vi "specify_roi.vi"(1 "input cluster":T3) -> (0 "output cluster":cluster{"Value":i32, dbl[], "Set":bool})   [LabVIEW 2015]
uses:
  <vilib>/vision/Avi1.llb/AviRefnum.ctl
  <vilib>/userdefined/High Color/IMAQdx.ctl
panel:
  in  "Store ROI from Coords":bool
  in  "Store ROI from image":bool
  in  "ROI Type":bool
  in  "ROI type flag":i32=-1
  in  "y2":i32
  in  "x2":i32
  in  "y1":i32
  in  "x1":i32
  out "initital frame number":i32
  in  "Reset":bool
  out "Image":T4(plugin-control)
  in  "Cancel":bool
  in  "Set":bool
  # "ROI Type"
  # "Rectangle"
  # "Ellipse"
  # "ROI Coordinates"
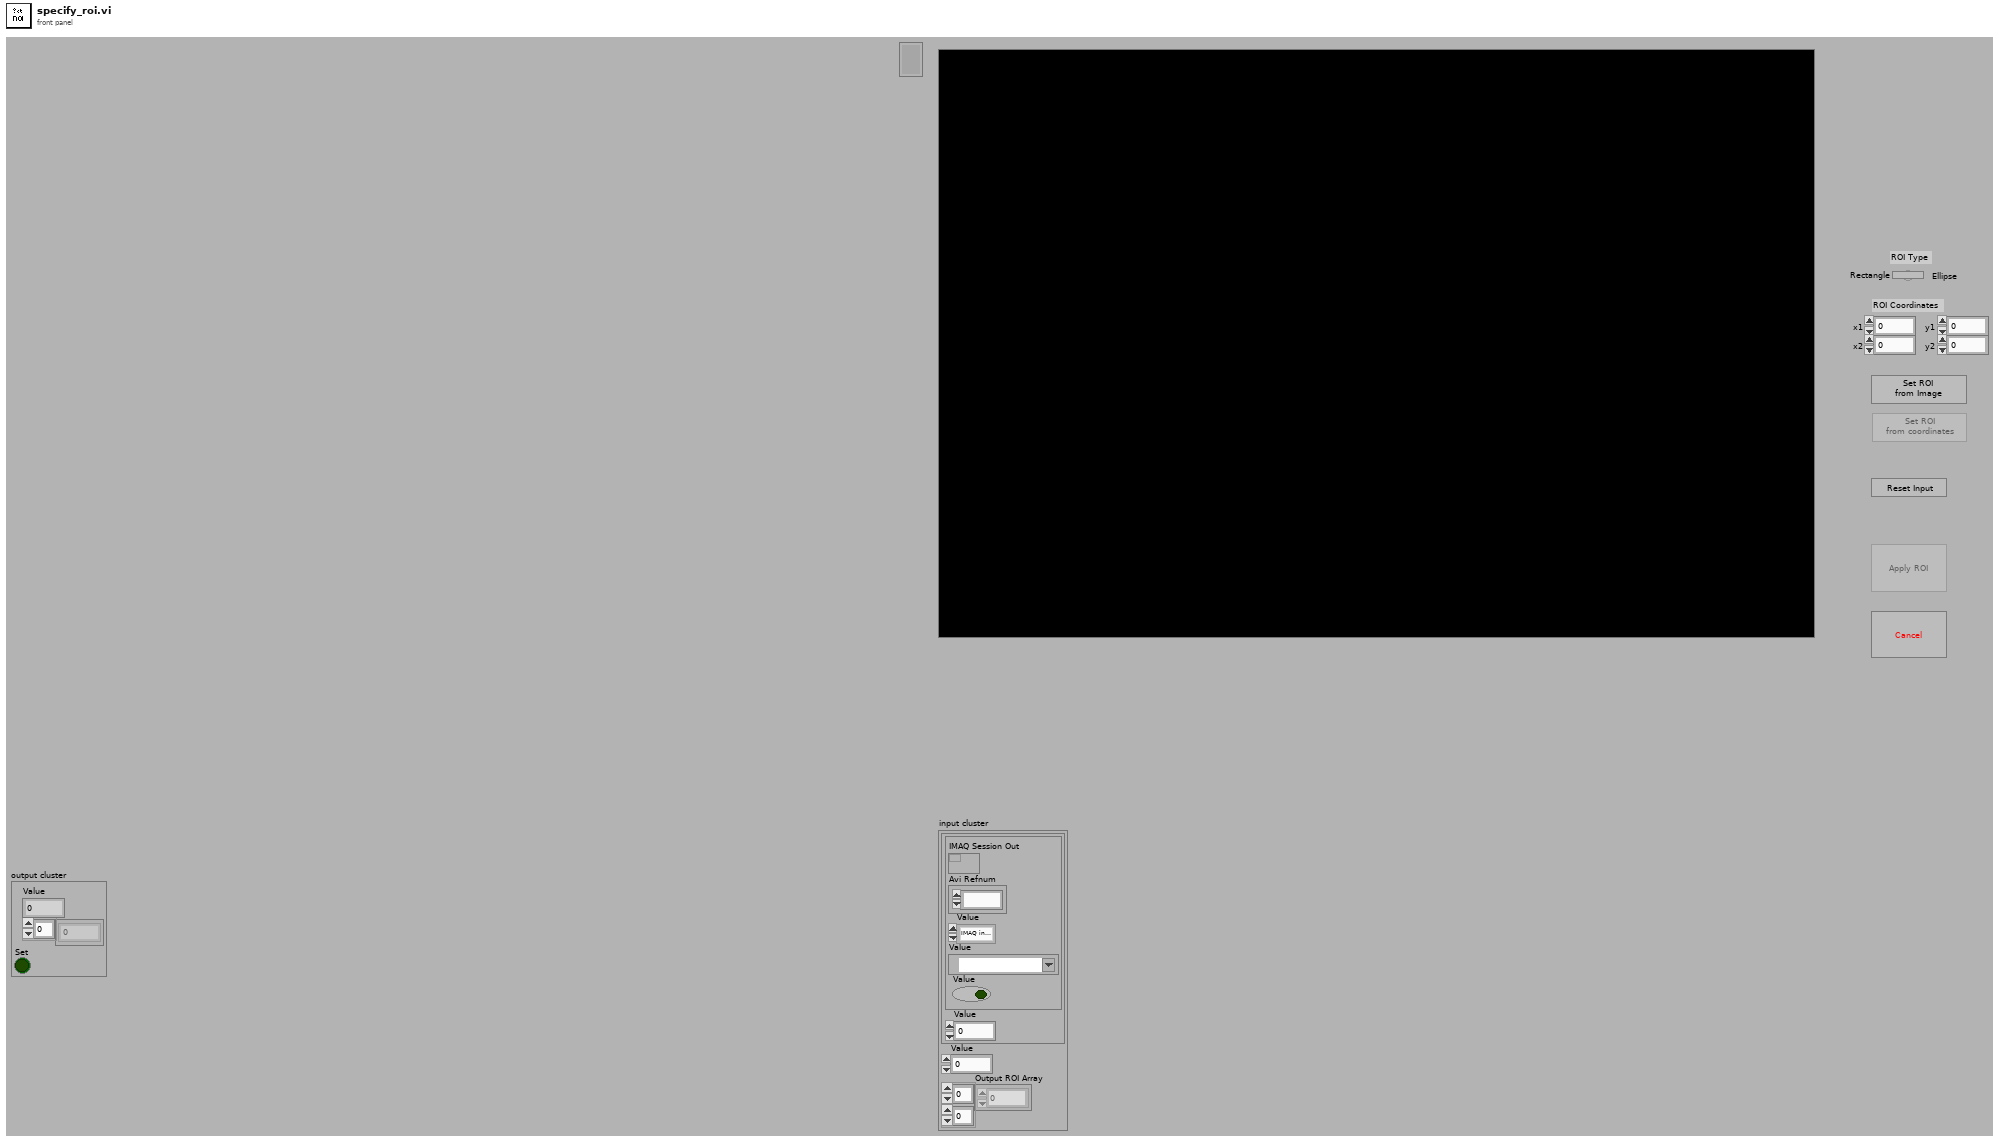
[diagram p1: front panel]
types:
  T1 = typedef "AviRefnum.ctl" = refnum<k1>
  T2 = typedef "IMAQdx.ctl" = refnum<k21>
  T3 = cluster{cluster{cluster{"IMAQ Session Out":refnum<k11>, "Avi Refnum":T1, "Value":enum32{"IMAQ interface", "IMAQdx interface", "AVI file"}, "Value":T2, "Value":bool}, "Value":i32}, "Value":i32, "Output ROI Array":dbl[][]}
  T4 = typedef "IMAQ Image.ctl" = refnum<image>
  T5 = cluster{cluster{"IMAQ Session Out":refnum<k11>, "Avi Refnum":T1, "Value":enum32{"IMAQ interface", "IMAQdx interface", "AVI file"}, "Value":T2, "Value":bool}, "Value":i32}
  T6 = cluster{"Global Rectangle":i32[], "Contours":cluster{"Contour Type":u32, "ROI Type":u32, "Points":i32[]}[]}
  T7 = enum8{"Enabled", "Disabled", "Disabled and Grayed Out"}
  T8 = cluster{"IMAQ Session Out":refnum<k11>, "Avi Refnum":T1, "Value":enum32{"IMAQ interface", "IMAQdx interface", "AVI file"}, "Value":T2, "Value":bool}
  T9 = cluster{cluster{"IMAQ Session Out":refnum<k11>, "Avi Refnum":T1, "Value":enum32{"IMAQ interface", "IMAQdx interface", "AVI file"}, "Value":T2, "Value":bool}, "Acquired Buffer Number":i32}
  T10 = cluster{"Contour Type":u32, "ROI Type":u32, "Points":i32[]}[]
  T11 = cluster{"Contour Type":u32, "ROI Type":u32, "Points":i32[]}
  T12 = cluster{"Contour Type":u32, u32, "Points":i32[]}[]
  T13 = cluster{"Global Rectangle":i32[], cluster{"Contour Type":u32, u32, "Points":i32[]}[]}
  T14 = cluster{"Value":i32, "Output ROI Array":dbl[][], "Value":bool, i32[], cluster{dbl, dbl}, "Image Area Size":cluster{"Width":u32, "Height":u32}, "Image Dst Out":T4, "Image Out":T4}
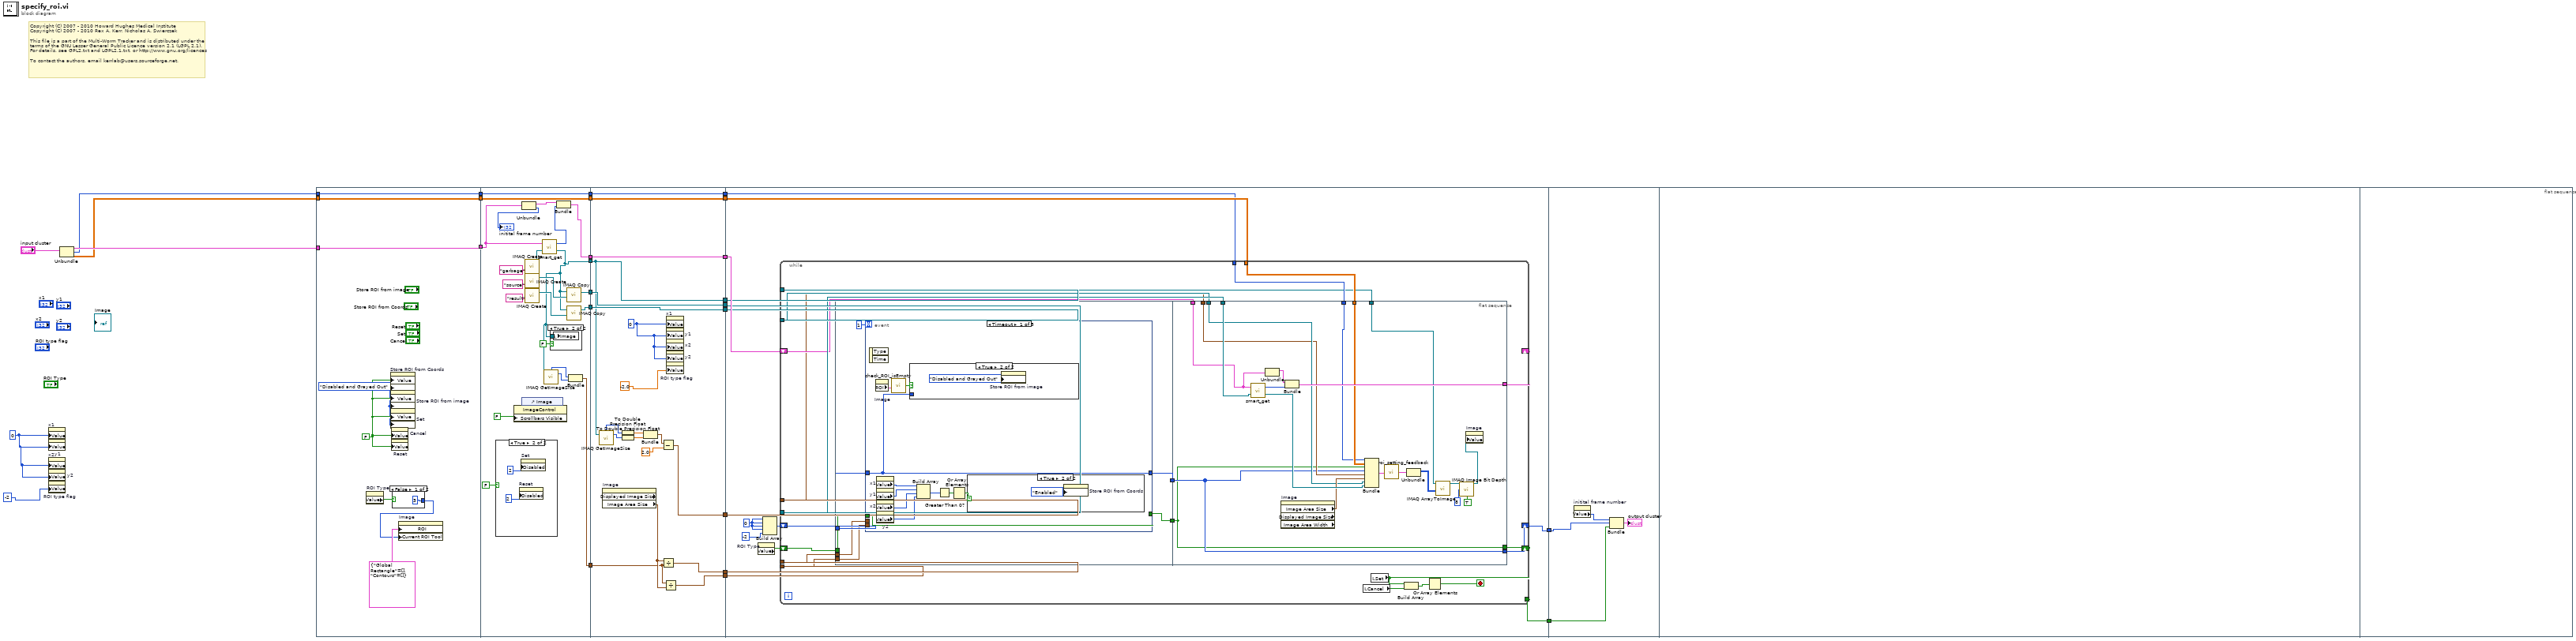
[diagram p0: block diagram]
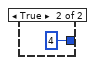
[diagram p2: hidden frame]
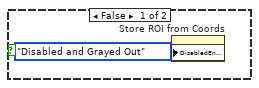
[diagram p5: hidden frame]
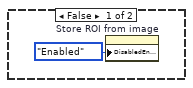
[diagram p6: hidden frame]
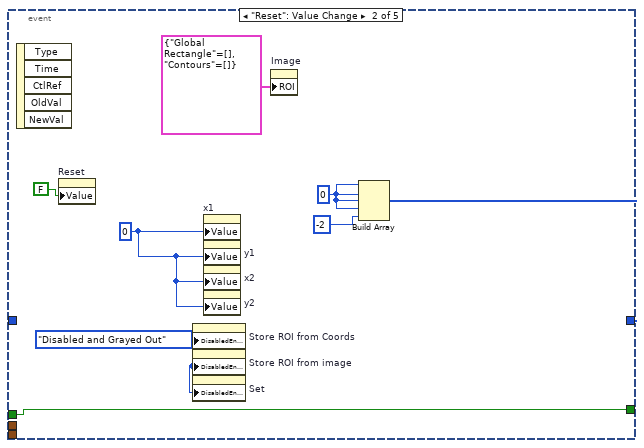
[diagram p7: hidden frame]
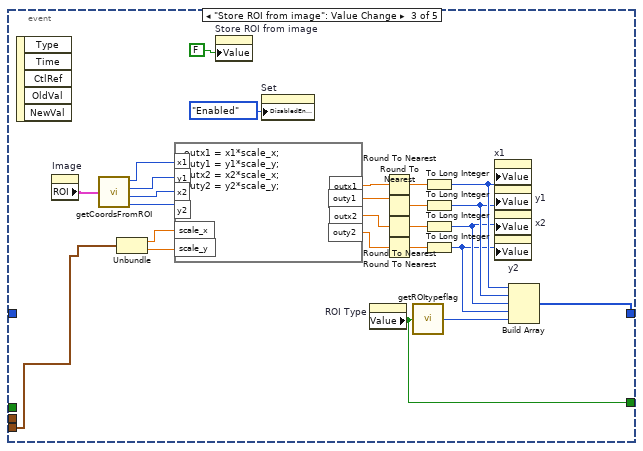
[diagram p8: hidden frame]
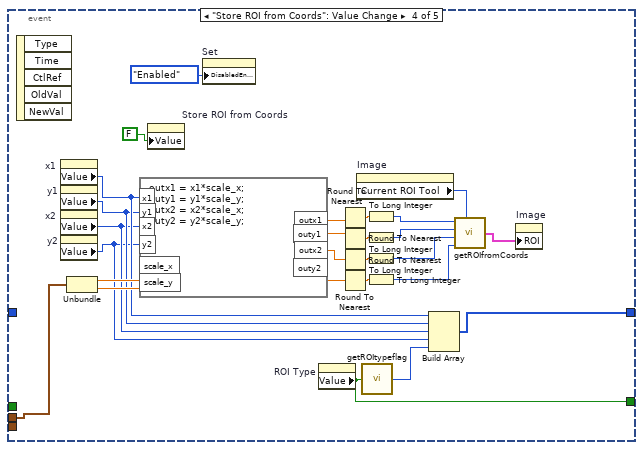
[diagram p9: hidden frame]
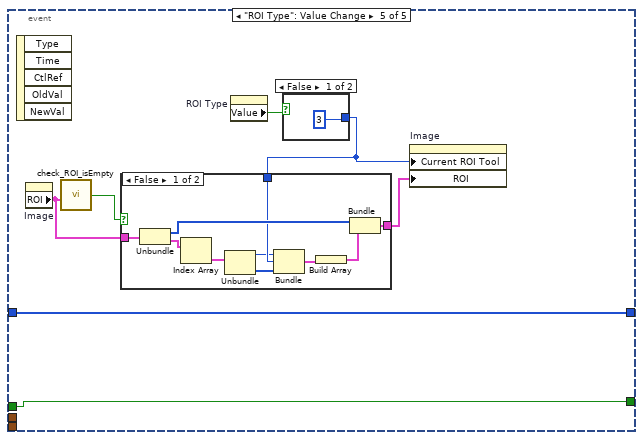
[diagram p10: hidden frame]
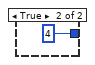
[diagram p12: hidden frame]
diagram:
  w7 = 0 ("x1")
  # "Copyright (C) 2007 - 2010 Howard Hughes Medical Institute\nCopyright (C) 2007 - 2010 Rex A. Kerr, Nicholas A. Swierczek\n \nThis file is a part of the Multi-Worm Tracker and is distributed under the\nterms of the GNU Lesser General Public Licence version 2.1 (LGPL 2.1).\nFor details, see GPL2.txt and LGPL2.1.txt, or http://www.gnu.org/licences\n \nTo contact the authors, email kerrlab@users.sourceforge.net."
  n1 = property on="x1" class="DigNum (strict)"("Value"=w7) -> ()  [unwired: 2 in, 2 out]
  n2 = property on="y1" class="DigNum (strict)"("Value"=w7) -> ()  [unwired: 2 in, 2 out]
  n3 = property on="x2" class="DigNum (strict)"("Value"=w7) -> ()  [unwired: 2 in, 2 out]
  n4 = property on="y2" class="DigNum (strict)"("Value"=w7) -> ()  [unwired: 2 in, 2 out]
  n5 = property on="ROI type flag" class="DigNum (strict)"("Value"=-2 ("x1")) -> ()  [unwired: 2 in, 2 out]
  n6 = Unbundle("input cluster") -> (w18:T5, "Value"=w17:i32, "Output ROI Array"=w16:dbl[][])
  n7 = flat-sequence {
    tunnel: [w34] -> w25
    tunnel: [w35] -> w23
    tunnel: w16 -> [w35]
    tunnel: w18 -> [w34]
    tunnel: [w33] -> w19
    tunnel: w17 -> [w33]
    tunnel: [w45] -> w27
    tunnel: [w42] -> w26
    tunnel: w25 -> [w46]
    tunnel: [w57] -> w24
    tunnel: w23 -> [w57]
    tunnel: [w53] -> w22
    tunnel: [w54] -> w21
    tunnel: [w49] -> w20
    tunnel: w19 -> [w49]
    tunnel: [w39] -> w6
    tunnel: [w70] -> w14
    tunnel: [w71] -> w13
    tunnel: [w72] -> w12
    tunnel: w27 -> [w78]
    tunnel: w26 -> [w70]
    tunnel: [w78] -> w11
    tunnel: [w74] -> w10
    tunnel: w24 -> [w74]
    tunnel: w22 -> [w72]
    tunnel: w21 -> [w71]
    tunnel: [w73] -> w9
    tunnel: w20 -> [w73]
    tunnel: [w75] -> w8
    tunnel: w6 -> [w65]
    tunnel: [w67] -> w3
    tunnel: [w64] -> w2
    tunnel: w14 -> [w91]
    tunnel: w13 -> [w92]
    tunnel: w12 -> [w93]
    tunnel: w11 -> [w97]
    tunnel: w10 -> [w95]
    tunnel: w9 -> [w94]
    tunnel: w8 -> [w96]
    tunnel: [w90] -> w5
    tunnel: [w89] -> w4
    tunnel: w3 -> [w85]
    tunnel: w2 -> [w84]
    tunnel: w5 -> [w241]
    tunnel: w4 -> [w240]
    frame #0 {
      w28 = T7."Disabled and Grayed Out" ("Disabled")
      w29 = FALSE ("Set")
      n8 = property on="ROI Type" class="Bool (strict)"() -> ("Value"=w31:bool)  [unwired: 2 in, 2 out]
      n9 = property on="Store ROI from Coords" class="Bool (strict)"("Value"=w29, "DisabledEnum"=w28) -> ()  [unwired: 2 in, 2 out]
      n10 = property on="Store ROI from image" class="Bool (strict)"("Value"=w29, "DisabledEnum"=w28) -> ()  [unwired: 2 in, 2 out]
      n11 = property on="Set" class="Bool (strict)"("Value"=w29, "DisabledEnum"=w28) -> ()  [unwired: 2 in, 2 out]
      n12 = property on="Cancel" class="Bool (strict)"("Value"=w29) -> ()  [unwired: 2 in, 2 out]
      n13 = property on="Reset" class="Bool (strict)"("Value"=w29) -> ()  [unwired: 2 in, 2 out]
      n14 = case shown="False" w31 {
        tunnel: [u32 3 u32 4] -> w30
        frame False {
        }
        frame True {
        }
      }
      n15 = property on="Image" class="ImageControl"("ROI"=T6 {"Global Rectangle"=[], "Contours"=[]}, "Current ROI Tool"=w30) -> ()  [unwired: 2 in, 2 out]
    }
    frame #1 {
      n16 = case shown="True" FALSE {
        frame False {
        }
        frame True {
          n17 = property on="Reset" class="Bool (strict)"("Disabled"=u8 2) -> ()  [unwired: 2 in, 2 out]
          n18 = property on="Set" class="Bool (strict)"("Disabled"=u8 2) -> ()  [unwired: 2 in, 2 out]
        }
      }
      n19 = Unbundle(w46) -> (w48:T8, "Value"=→"initital frame number":i32)
      n20 = control-ref of="Image"() -> (w60:refnum<vi>)
      n21 = property class="ImageControl"(reference=w60, "Scrollbars Visible"=FALSE) -> ()  [unwired: 1 in, 2 out]
      n22 = call "IMAQ Create"("Image Name"="garbage") -> ("New Image"=w50:T4)  [unwired: 4 in, 1 out]
      n23 = call "IMAQ Create"("Image Name"="source") -> ("New Image"=w52:T4)  [unwired: 4 in, 1 out]
      n24 = call "IMAQ Create"("Image Name"="result") -> ("New Image"=w51:T4)  [unwired: 4 in, 1 out]
      n25 = call "smart_get.vi"("Input Image"=w50, "Cluster"=w46) -> ("Image Out"=w42:T4, "Acquired Buffer Number"=w47:i32)
      n26 = call "IMAQ GetImageSize"("Image"=w42) -> ("Y Resolution"=w41:i32, "X Resolution"=w40:i32)  [unwired: 3 in, 1 out]
      n27 = case shown="True" FALSE {
        tunnel: w42 -> [_ w61]
        frame False {
        }
        frame True {
          n28 = local write "Image"(w61) -> ()
        }
      }
      n29 = Bundle(w48, "Acquired Buffer Number"=w47) -> (w45:T9)  [unwired: 1 in]
      n30 = call "IMAQ Copy"("Image Dst"=w52, "Image Src"=w42) -> ("Image Dst Out"=w53:T4)  [unwired: 4 in, 1 out]
      n31 = call "IMAQ Copy"("Image Dst"=w51, "Image Src"=w42) -> ("Image Dst Out"=w54:T4)  [unwired: 4 in, 1 out]
      n32 = Bundle("X Resolution"=w40, "Y Resolution"=w41) -> (w39:cluster{"X Resolution":i32, "Y Resolution":i32})  [unwired: 1 in]
    }
    frame #2 {
      w69 = 0 ("x1")
      n33 = call "IMAQ GetImageSize"("Image"=w70) -> ("Y Resolution"=w81:i32, "X Resolution"=w82:i32)  [unwired: 3 in, 1 out]
      n34 = property on="Image" class="ImageControl" props=["Displayed Image Size", "Image Area Size"]() -> ("Image Area Size"=w66:cluster{"Width":u32, "Height":u32})  [unwired: 2 in, 3 out]
      n35 = To Double Precision Float(number=w82) -> (double precision float=w80:dbl)
      n36 = To Double Precision Float(number=w81) -> (double precision float=w79:dbl)
      n37 = Bundle(w80, w79) -> (w76:cluster{dbl, dbl})  [unwired: 1 in]
      n38 = Subtract(x=w76, y=2.0) -> (x-y=w75:cluster{dbl, dbl})
      n39 = Divide(x=w66, y=w65) -> (x/y=w67:cluster{dbl, dbl})
      n40 = Divide(x=w65, y=w66) -> (x/y=w64:cluster{dbl, dbl})
      n41 = property on="x1" class="DigNum (strict)"("Value"=w69) -> ()  [unwired: 2 in, 2 out]
      n42 = property on="y1" class="DigNum (strict)"("Value"=w69) -> ()  [unwired: 2 in, 2 out]
      n43 = property on="x2" class="DigNum (strict)"("Value"=w69) -> ()  [unwired: 2 in, 2 out]
      n44 = property on="y2" class="DigNum (strict)"("Value"=w69) -> ()  [unwired: 2 in, 2 out]
      n45 = property on="ROI type flag" class="DigNum (strict)"("Value"=-2.0 ("x1")) -> ()  [unwired: 2 in, 2 out]
    }
    frame #3 {
      w88 = 0 ("x1")
      n46 = property on="ROI Type" class="Bool (strict)"() -> ("Value"=w83:bool)  [unwired: 2 in, 2 out]
      n47 = Build Array(w88, w88, w88, w88, -2 ("x1")) -> (w86:i32[])
      n48 = while {
        shift-right: [w113] -> _
        shift-left: w97 -> [w109]
        tunnel: w96 -> [w106]
        tunnel: w95 -> [w111]
        tunnel: w94 -> [w108]
        tunnel: w93 -> [w110]
        tunnel: w92 -> [w107]
        tunnel: w91 -> [w105]
        tunnel: [w114] -> w89
        shift-right: [w103] -> w90
        shift-left: w86 -> [w112]
        tunnel: w85 -> [w102]
        shift-right: [w98] -> _
        shift-left: w83 -> [w100]
        tunnel: w84 -> [w101]
        stop <- w115 stop-if-true
        n49 = flat-sequence {
          tunnel: w112 -> [w123]
          tunnel: [w122] -> w104
          tunnel: w102 -> [w121]
          tunnel: w101 -> [w120]
          tunnel: w100 -> [w119]
          tunnel: [w118] -> w99
          tunnel: [w239] -> w113
          tunnel: w111 -> [w229]
          tunnel: w108 -> [w228]
          tunnel: w110 -> [w227]
          tunnel: w109 -> [w226]
          tunnel: w107 -> [w225]
          tunnel: w106 -> [w224]
          tunnel: w105 -> [w223]
          tunnel: w104 -> [w220]
          tunnel: [w220] -> w103
          tunnel: w99 -> [w219]
          tunnel: [w219] -> w98
          frame #0 {
            n50 = event shown="[0] Timeout" {
              selector: _ -> [_ _ _ _ _]
              dyn-events: _ -> [_ _ _ _ _]
              timeout: 1 -> [_ _ _ _ _]
              tunnel: w123 -> [w133 _ _ _ w205]
              tunnel: [w133 w141 w171 w197 w205] -> w122
              tunnel: w121 -> [_ _ _ w198 _]
              tunnel: w120 -> [_ _ w172 _ _]
              tunnel: w119 -> [w125 w140 _ _ w203]
              tunnel: [w125 w140 w148 w177 w203] -> w118
              event Timeout {
                n51 = event-data() -> ()  [unwired: 1 in, 2 out]
                n52 = property on="Image" class="ImageControl"() -> ("ROI"=w135:T6)  [unwired: 2 in, 2 out]
                n53 = property on="x1" class="DigNum (strict)"() -> ("Value"=w132:i32)  [unwired: 2 in, 2 out]
                n54 = property on="y1" class="DigNum (strict)"() -> ("Value"=w131:i32)  [unwired: 2 in, 2 out]
                n55 = property on="x2" class="DigNum (strict)"() -> ("Value"=w130:i32)  [unwired: 2 in, 2 out]
                n56 = property on="y2" class="DigNum (strict)"() -> ("Value"=w129:i32)  [unwired: 2 in, 2 out]
                n57 = call "check_ROI_isEmpty.vi"("ROI"=w135) -> ("empty?"=w134:bool)
                n58 = case shown="True" w134 {
                  tunnel: w133 -> [_ _]
                  frame False {
                    n59 = property on="Store ROI from image" class="Bool (strict)"("DisabledEnum"=T7."Enabled" ("Disabled")) -> ()  [unwired: 2 in, 2 out]
                  }
                  frame True {
                    n60 = property on="Store ROI from image" class="Bool (strict)"("DisabledEnum"=T7."Disabled and Grayed Out" ("Disabled")) -> ()  [unwired: 2 in, 2 out]
                  }
                }
                n61 = Build Array(w132, w131, w130, w129) -> (w128:i32[])
                n62 = Greater Than 0?(x=w128) -> (x > 0?=w127:bool[])
                n63 = Or Array Elements(Boolean array=w127) -> (logical OR=w126:bool)
                n64 = case shown="True" w126 {
                  frame False {
                    n65 = property on="Store ROI from Coords" class="Bool (strict)"("DisabledEnum"=T7."Disabled and Grayed Out" ("Disabled")) -> ()  [unwired: 2 in, 2 out]
                  }
                  frame True {
                    n66 = property on="Store ROI from Coords" class="Bool (strict)"("DisabledEnum"=T7."Enabled" ("Disabled")) -> ()  [unwired: 2 in, 2 out]
                  }
                }
              }
              event "Reset": Value Change {
                w142 = 0 ("x1")
                w144 = T7."Disabled and Grayed Out" ("Disabled")
                w146 = 0 ("x1")
                n67 = event-data() -> ()  [unwired: 1 in, 5 out]
                n68 = property on="Reset" class="Bool (strict)"("Value"=FALSE ("Set")) -> ()  [unwired: 2 in, 2 out]
                n69 = property on="Store ROI from Coords" class="Bool (strict)"("DisabledEnum"=w144) -> ()  [unwired: 2 in, 2 out]
                n70 = property on="Store ROI from image" class="Bool (strict)"("DisabledEnum"=w144) -> ()  [unwired: 2 in, 2 out]
                n71 = property on="Set" class="Bool (strict)"("DisabledEnum"=w144) -> ()  [unwired: 2 in, 2 out]
                n72 = property on="x1" class="DigNum (strict)"("Value"=w146) -> ()  [unwired: 2 in, 2 out]
                n73 = property on="y1" class="DigNum (strict)"("Value"=w146) -> ()  [unwired: 2 in, 2 out]
                n74 = property on="x2" class="DigNum (strict)"("Value"=w146) -> ()  [unwired: 2 in, 2 out]
                n75 = property on="y2" class="DigNum (strict)"("Value"=w146) -> ()  [unwired: 2 in, 2 out]
                n76 = property on="Image" class="ImageControl"("ROI"=T6 {"Global Rectangle"=[], "Contours"=[]}) -> ()  [unwired: 2 in, 2 out]
                n77 = Build Array(w142, w142, w142, w142, -2 ("x1")) -> (w141:i32[])
              }
              event "Store ROI from image": Value Change {
                n78 = event-data() -> ()  [unwired: 1 in, 5 out]
                n79 = property on="Image" class="ImageControl"() -> ("ROI"=w170:T6)  [unwired: 2 in, 2 out]
                n80 = call "getCoordsFromROI.vi"("ROI"=w170) -> ("y2"=w166:i32, "x2"=w167:i32, "y1"=w168:i32, "x1"=w169:i32)
                n81 = Unbundle(w172) -> (w165:dbl, w164:dbl)
                n82 = formula code="outx1 = x1*scale_x;\nouty1 = y1*scale_y;\noutx2 = x2*scale_x;\nouty2 = y2*scale_y;"("x1"=w169, "y1"=w168, "x2"=w167, "y2"=w166, "scale_x"=w165, "scale_y"=w164) -> ("outx1"=w163:dbl, "outy1"=w162:dbl, "outx2"=w161:dbl, "outy2"=w160:dbl)
                n83 = property on="Store ROI from image" class="Bool (strict)"("Value"=FALSE ("Set")) -> ()  [unwired: 2 in, 2 out]
                n84 = property on="Set" class="Bool (strict)"("DisabledEnum"=T7."Enabled" ("Disabled")) -> ()  [unwired: 2 in, 2 out]
                n85 = property on="ROI Type" class="Bool (strict)"() -> ("Value"=w148:bool)  [unwired: 2 in, 2 out]
                n86 = Round To Nearest(number=w163) -> (nearest integer value=w159:dbl)
                n87 = Round To Nearest(number=w162) -> (nearest integer value=w158:dbl)
                n88 = Round To Nearest(number=w161) -> (nearest integer value=w157:dbl)
                n89 = Round To Nearest(number=w160) -> (nearest integer value=w156:dbl)
                n90 = call "getROItypeflag.vi"("ROI type"=w148) -> ("ROI Type flag"=w154:i32)
                n91 = To Long Integer(number=w159) -> (32bit integer=w153:i32)
                n92 = To Long Integer(number=w158) -> (32bit integer=w152:i32)
                n93 = To Long Integer(number=w157) -> (32bit integer=w151:i32)
                n94 = To Long Integer(number=w156) -> (32bit integer=w150:i32)
                n95 = property on="x1" class="DigNum (strict)"("Value"=w153) -> ()  [unwired: 2 in, 2 out]
                n96 = property on="y1" class="DigNum (strict)"("Value"=w152) -> ()  [unwired: 2 in, 2 out]
                n97 = property on="x2" class="DigNum (strict)"("Value"=w151) -> ()  [unwired: 2 in, 2 out]
                n98 = property on="y2" class="DigNum (strict)"("Value"=w150) -> ()  [unwired: 2 in, 2 out]
                n99 = Build Array(w153, w152, w151, w150, w154) -> (w171:i32[])
              }
              event "Store ROI from Coords": Value Change {
                n100 = event-data() -> ()  [unwired: 1 in, 5 out]
                n101 = property on="x1" class="DigNum (strict)"() -> ("Value"=w176:i32)  [unwired: 2 in, 2 out]
                n102 = property on="y1" class="DigNum (strict)"() -> ("Value"=w175:i32)  [unwired: 2 in, 2 out]
                n103 = property on="x2" class="DigNum (strict)"() -> ("Value"=w174:i32)  [unwired: 2 in, 2 out]
                n104 = property on="y2" class="DigNum (strict)"() -> ("Value"=w173:i32)  [unwired: 2 in, 2 out]
                n105 = Unbundle(w198) -> (w196:dbl, w195:dbl)
                n106 = formula code="outx1 = x1*scale_x;\nouty1 = y1*scale_y;\noutx2 = x2*scale_x;\nouty2 = y2*scale_y;"("x1"=w176, "y1"=w175, "x2"=w174, "y2"=w173, "scale_x"=w196, "scale_y"=w195) -> ("outx1"=w194:dbl, "outy1"=w193:dbl, "outx2"=w192:dbl, "outy2"=w191:dbl)
                n107 = property on="Store ROI from Coords" class="Bool (strict)"("Value"=FALSE ("Set")) -> ()  [unwired: 2 in, 2 out]
                n108 = property on="Set" class="Bool (strict)"("DisabledEnum"=T7."Enabled" ("Disabled")) -> ()  [unwired: 2 in, 2 out]
                n109 = property on="ROI Type" class="Bool (strict)"() -> ("Value"=w177:bool)  [unwired: 2 in, 2 out]
                n110 = Round To Nearest(number=w194) -> (nearest integer value=w190:dbl)
                n111 = Round To Nearest(number=w193) -> (nearest integer value=w189:dbl)
                n112 = Round To Nearest(number=w192) -> (nearest integer value=w188:dbl)
                n113 = Round To Nearest(number=w191) -> (nearest integer value=w187:dbl)
                n114 = property on="Image" class="ImageControl"() -> ("Current ROI Tool"=w184:u32)  [unwired: 2 in, 2 out]
                n115 = call "getROItypeflag.vi"("ROI type"=w177) -> ("ROI Type flag"=w179:i32)
                n116 = To Long Integer(number=w190) -> (32bit integer=w183:i32)
                n117 = To Long Integer(number=w189) -> (32bit integer=w182:i32)
                n118 = To Long Integer(number=w188) -> (32bit integer=w181:i32)
                n119 = To Long Integer(number=w187) -> (32bit integer=w180:i32)
                n120 = Build Array(w176, w175, w174, w173, w179) -> (w197:i32[])
                n121 = call "getROIfromCoords.vi"("x1"=w183, "y1"=w182, "x2"=w181, "y2"=w180, "type"=w184) -> ("ROI"=w185:T6)
                n122 = property on="Image" class="ImageControl"("ROI"=w185) -> ()  [unwired: 2 in, 2 out]
              }
              event "ROI Type": Value Change {
                n123 = event-data() -> ()  [unwired: 1 in, 5 out]
                n124 = property on="Image" class="ImageControl"() -> ("ROI"=w201:T6)  [unwired: 2 in, 2 out]
                n125 = call "check_ROI_isEmpty.vi"("ROI"=w201) -> ("empty?"=w202:bool)
                n126 = property on="ROI Type" class="Bool (strict)"() -> ("Value"=w204:bool)  [unwired: 2 in, 2 out]
                n127 = case shown="False" w204 {
                  tunnel: [u32 3 u32 4] -> w200
                  frame False {
                  }
                  frame True {
                  }
                }
                n128 = case shown="False" w202 {
                  tunnel: w201 -> [w215 w216]
                  tunnel: w200 -> [w211 _]
                  tunnel: [w206 w216] -> w199
                  frame False {
                    n129 = Unbundle(w215) -> ("Global Rectangle"=w214:i32[], "Contours"=w213:T10)
                    n130 = Index Array(array=w213) -> (element=w212:T11)  [unwired: 1 in]
                    n131 = Unbundle(w212) -> ("Contour Type"=w210:u32, "Points"=w209:i32[])  [unwired: 1 out]
                    n132 = Bundle("Contour Type"=w210, w211, "Points"=w209) -> (w208:cluster{"Contour Type":u32, u32, "Points":i32[]})  [unwired: 1 in]
                    n133 = Build Array(w208) -> (w207:T12)
                    n134 = Bundle("Global Rectangle"=w214, w207) -> (w206:T13)  [unwired: 1 in]
                  }
                  frame True {
                    # "Do nothing."
                  }
                }
                n135 = property on="Image" class="ImageControl"("Current ROI Tool"=w200, "ROI"=w199) -> ()  [unwired: 2 in, 2 out]
              }
            }
          }
          frame #1 {
            n136 = call "smart_get.vi"("Input Image"=w227, "Cluster"=w226) -> ("Image Out"=w238:T4, "Acquired Buffer Number"=w236:i32)
            n137 = Unbundle(w226) -> (w237:T8)  [unwired: 1 out]
            n138 = property on="Image" class="ImageControl" props=["Image Area Size", "Displayed Image Size", "Image Area Width"]() -> ("Image Area Size"=w235:cluster{"Width":u32, "Height":u32})  [unwired: 2 in, 4 out]
            n139 = Bundle(w237, "Acquired Buffer Number"=w236) -> (w239:T9)  [unwired: 1 in]
            n140 = Bundle("Value"=w228, "Output ROI Array"=w229, "Value"=w219, w220, w224, "Image Area Size"=w235, "Image Dst Out"=w225, "Image Out"=w238) -> (w221:T14)  [unwired: 1 in]
            n141 = call "roi_setting_feedback.vi"("input cluster"=w221) -> ("output cluster"=w233:cluster{"destination":i16[][], dbl[]})
            n142 = Unbundle(w233) -> ("destination"=w234:i16[][])  [unwired: 1 out]
            n143 = call "IMAQ ArrayToImage"("Image Pixels (I16)"=w234, "Image"=w223) -> ("Image Out"=w231:T4)  [unwired: 8 in, 1 out]
            n144 = call "IMAQ Image Bit Depth"("Image"=w231, "Bit Depth (0)"=u32 8, "Get/Set Bit Depth? (Set)"=TRUE) -> ("Image Out"=w222:T4)  [unwired: 10 in, 2 out]
            n145 = property on="Image" class="ImageControl"("Value"=w222) -> ()  [unwired: 2 in, 2 out]
          }
        }
        n146 = local read "Cancel"() -> (w116:bool)
        n147 = local read "Set"() -> (w114:bool)
        n148 = Build Array(w114, w116) -> (w117:bool[])
        n149 = Or Array Elements(Boolean array=w117) -> (logical OR=w115:bool)
      }
    }
    frame #4 {
      n150 = property on="initital frame number" class="DigNum (strict)"() -> ("Value"=w242:i32)  [unwired: 2 in, 2 out]
      n151 = Bundle("Value"=w242, w241, "Set"=w240) -> (→"output cluster":cluster{"Value":i32, i32[], "Set":bool})  [unwired: 1 in]
    }
    frame #5 {
    }
    frame #6 {
    }
  }
